vi "试验配置信息.vi"() -> ()   [LabVIEW 2010]
panel:
  in  "配置文件序号":u16
  out "D_IN_4":string[][](table) caption="表格"
  out "D_IN_3":string[][](table) caption="表格"
  out "D_IN_2":string[][](table) caption="表格"
  out "D_IN_1":string[][](table) caption="表格"
  out "板卡II自动检测结果":bool[](array[boolean])
  in  "自测类型4路数":i32
  in  "自测类型3路数":i32
  in  "自测类型2路数":i32
  in  "自测类型1路数":i32
  in  "测试类型4选择？":bool
  in  "测试类型3选择？":bool
  in  "测试类型2选择？":bool
  in  "测试类型1选择？":bool
  out "自动检测结果":bool[](array[boolean])
  in  "允许误差":dbl[](array[numeric])
  in  "跳变方向":i32[](array[numeric])
  in  "延时T":i32[](array[numeric])
  in  "Max":dbl[](array[numeric])
  in  "min":dbl[](array[numeric])
  in  "参数A3":dbl[](array[numeric])
  in  "参数A2":dbl[](array[numeric])
  in  "参数A1":dbl[](array[numeric])
  in  "输入切换ID":i32[](array[numeric])
  in  "输出切换ID":i32[](array[numeric])
  in  "设定输入通道":i32[](array[numeric])
  in  "设定输出通道":i32[](array[numeric])
  in  "名称":string[](array[string])
  in  "LAN选择？":bool
  in  "RS485选择？":bool
  in  "RS232选择？":bool
  in  "CAN选择？":bool
  in  "AD输入选择？":bool
  in  "DSP输入选择？":bool
  in  "数字量输出选择？":bool
  in  "数字量输入选择？":bool
  in  "自测LAN路数":i32
  in  "自测项数":i32
  in  "自测类数":i32
  in  "自测AI_DSP路数":i32
  in  "自测485路数":i32
  in  "自测RS232路数":i32
  in  "自测CAN路数":i32
  in  "自测AI_AD路数":i32
  in  "自测DO路数":i32
  in  "自测DI路数":i32
  in  "报告编号":string
  in  "测试地点":string
  in  "测试人员":string
  in  "控制板编号":string
  in  "控制板类型":string
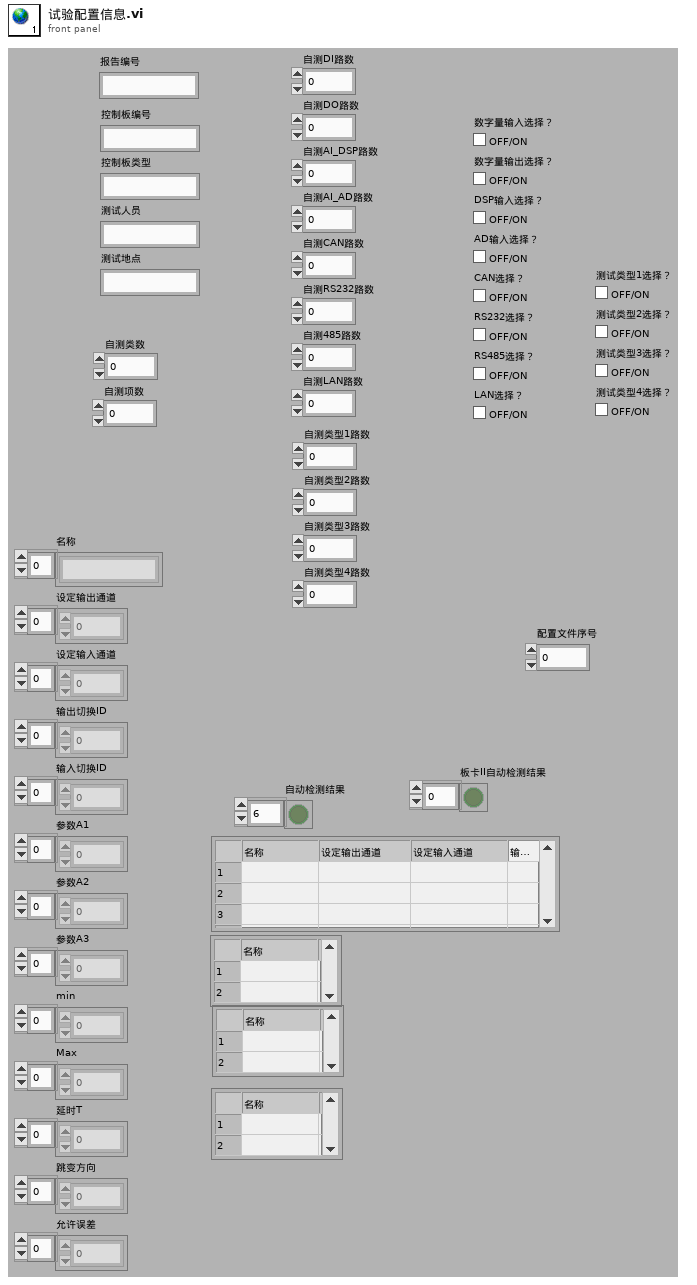
[diagram p1: front panel]
diagram:
